vi "Read BundleDefinition.vi"(8 "error in (no error)":errorcluster, 11 "Bundle Builder in":refnum<class "Bundle Builder.lvclass">) -> (0 "error out":errorcluster, 2 "BundleDefinition":refnum<k24>, 3 "Bundle Builder out":refnum<class "Bundle Builder.lvclass">)   [LabVIEW 2020]
uses:
  Bundle Builder.lvclass
  C:/Users/chihong/Documents/Repos/StsCustomBundleBuilder/Code/StsCustomBundleBuilderLib/StsCustomBundleBuilderLib/bin/Debug/StsCustomBundleBuilderLib.dll
  StsCustomBundleBuilderLib/StsCustomBundleBuilderLib/bin/Debug/StsCustomBundleBuilderLib.dll
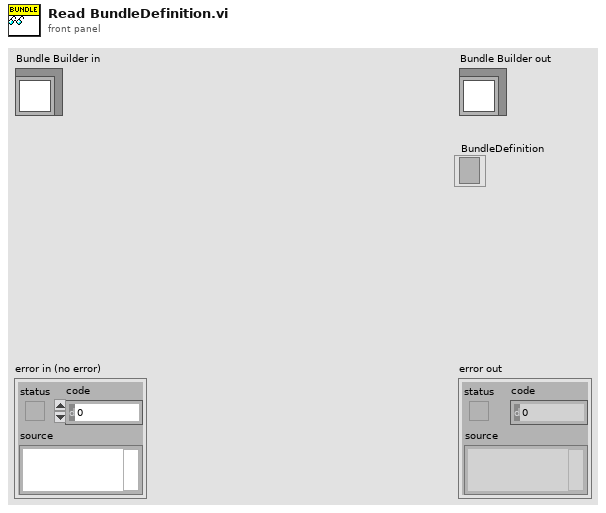
[diagram p1: front panel]
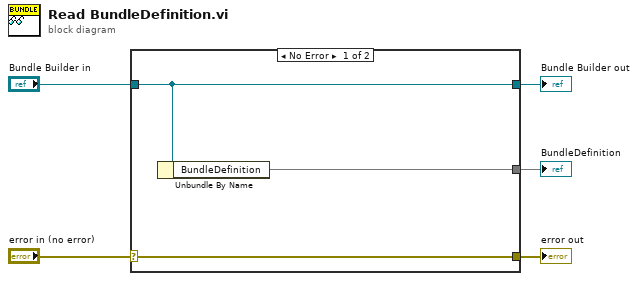
[diagram p0: block diagram]
diagram:
  n1 = case shown="No Error" "error in (no error)" {
    selector: "error in (no error)" -> [w8 w9]
    tunnel: [w8 w9] -> w4
    tunnel: [w7 w10] -> w2
    tunnel: "Bundle Builder in" -> [w7 w10]
    tunnel: [w6 _] -> w1
    frame No Error {
      n2 = Unbundle By Name(w7) -> ("BundleDefinition"=w6)
    }
    frame Error {
    }
  }
  "error out" <- w4
  "Bundle Builder out" <- w2
  "BundleDefinition" <- w1
